vi "LuaVIEW Register Private Function.vi"(5 "LuaVIEW reference in":T1, 7 "function VI path":path, 11 "error in (no error)":errorcluster) -> (6 "LuaVIEW reference out":T1, 15 "error out":errorcluster)   [LabVIEW 2012]
doc: "Open a reference to a LuaVIEW function VI and add it to the LuaVIEW state's private registry so that any script running under that state can call the function."
uses:
  typedefs/t_LuaVIEW Reference.ctl
  typedefs/et_LuaVIEW CIN Actions.ctl
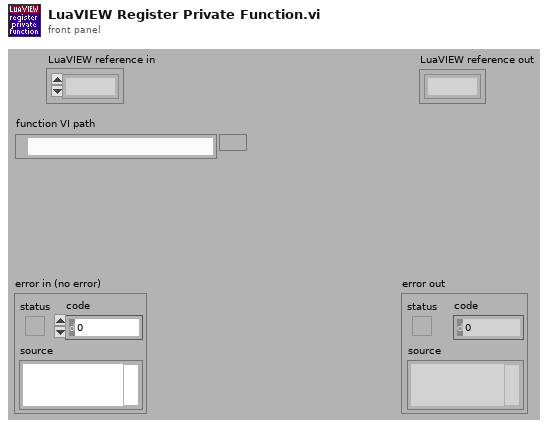
[diagram p1: front panel]
types:
  T1 = typedef "t_LuaVIEW Reference.ctl" = refnum<k1>
  T2 = typedef "et_LuaVIEW CIN Actions.ctl" = enum16{"checksynopsis", "_open", "_registerpublic", "_registerexport", "__never_an_error_result_ns", "luaversion", "cinversion", "_totals", "_taskcount", "pathological", "_unregnextpublic", "registryusecount", "__per_state_actions", "regsetprivate", "regsetindex", "regsetmodule", "_revokeexports", "_usepublic", "prepare", "compile", "execute", "call", "unregstaterefs", "_close", "pullboolean", "pullnumber", "pullI8", "pullU8", "pullI16", "pullU16", "pullI32", "pullU32", "pullobject", "pullrefnum", "pullstring", "pullflat", "pushflat", "pushobject", "getattribute", "setattribute", "stacktostring", "_startyieldtest", "_endyieldtest", "_pollprintbuffer", "__never_an_error_result_ps", "_pollexport", "setclone", "forcecleanup", "gettop", "clearstack", "insert", "pushboolean", "pushnumber", "pushrefnum", "pushstring", "pushnil", "pushvalue", "gettaskref", "settaskref"}
  T3 = typedef "et_LuaVIEW CIN Results.ctl" = enum16{"OK", "error", "main", "call", "clonecall", "modulecall", "exportcall", "index", "yield"}
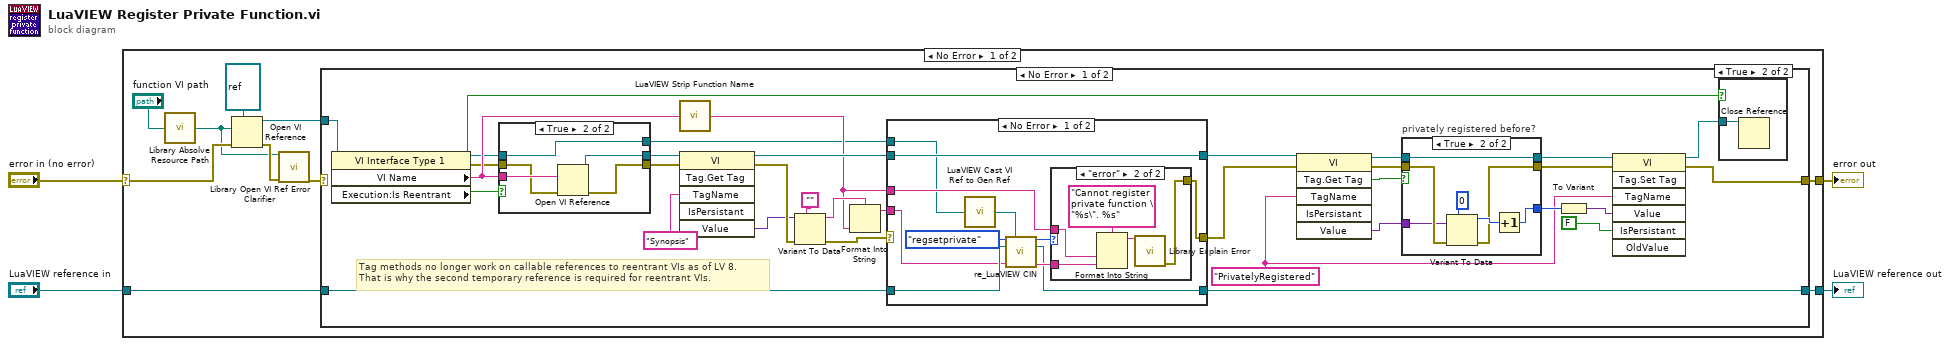
[diagram p0: block diagram]
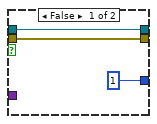
[diagram p4: hidden frame]
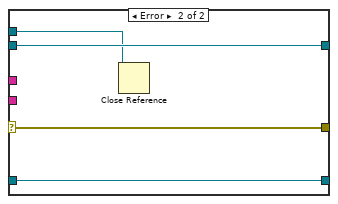
[diagram p6: hidden frame]
diagram:
  n1 = case shown="No Error" "error in (no error)" {
    selector: "error in (no error)" -> [w12 w89]
    tunnel: [w11 w89] -> w4
    tunnel: "LuaVIEW reference in" -> [w10 w88]
    tunnel: [w9 w88] -> w1
    frame No Error {
      n2 = call "Library Absolve Resource Path.vi"("path in"="function VI path") -> ("absolved path"=w7:path)  [unwired: 14 in]
      n3 = Open VI Reference(type specifier VI Refnum (for type only)=refnum<vi> refnum ("function pane"), vi path=w7, error in (no error)=w12) -> (vi reference=w6:refnum<vi>, error out=w8:errorcluster)  [unwired: 3 in]
      n4 = call "Library Open VI Ref Error Clarifier.vi"("VI path"=w7, "called VI error (no error)"=w8) -> ("error out"=w5:errorcluster)  [unwired: 13 in]
      n5 = case shown="No Error" w5 {
        selector: w5 -> [_ w87]
        tunnel: w6 -> [w23 _]
        tunnel: [w16 w87] -> w11
        tunnel: w10 -> [w45 w86]
        tunnel: [w44 w86] -> w9
        frame No Error {
          w35 = "PrivatelyRegistered"
          # "Tag methods no longer work on callable references to reentrant VIs as of LV 8.\nThat is why the second temporary reference is required for reentrant VIs."
          n6 = property class="VI Interface Type 1"(reference=w23) -> (reference out=w18:refnum<vi>, error out=w20:errorcluster, "VI Name"=w22:string, "Execution:Is Reentrant"=w15:bool)  [unwired: 1 in]
          n7 = case shown="True" w15 {
            tunnel: w22 -> [_ w54]
            tunnel: [w48 w53] -> w21
            tunnel: [w49 w51] -> w19
            tunnel: w20 -> [w49 w52]
            tunnel: w18 -> [w48 w50]
            tunnel: [w48 w50] -> w17
            frame False {
            }
            frame True {
              n8 = Open VI Reference(vi path=w54, error in (no error)=w52) -> (vi reference=w53:refnum<vi>, error out=w51:errorcluster)  [unwired: 4 in]
            }
          }
          n9 = call "LuaVIEW Strip Function Name.vi"("function VI name"=w22) -> ("Lua function name"=w24:string)  [unwired: 14 in]
          n10 = invoke class="VI" method="Tag.Get Tag"(reference=w21, error in=w19, "TagName"="Synopsis") -> (reference out=w27:refnum<vi>, error out=w32:errorcluster, "Value"=w28:variant)  [unwired: 3 in, 3 out]
          n11 = Variant To Data(error in=w32, type="", Variant=w28) -> (data=w29:string, error out=w25:errorcluster)
          n12 = Format Into String(format string=w29, w24) -> (resulting string=w26:string)  [unwired: 2 in, 1 out]
          n13 = case shown="No Error" w25 {
            selector: w25 -> [_ w84]
            tunnel: w45 -> [w74 w85]
            tunnel: [w71 w85] -> w44
            tunnel: w27 -> [w67 w83]
            tunnel: w26 -> [w70 _]
            tunnel: w24 -> [w69 _]
            tunnel: [w68 w84] -> w34
            tunnel: [w67 w83] -> w39
            tunnel: w17 -> [w66 w82]
            frame No Error {
              n14 = call "LuaVIEW Cast VI Ref to Gen Ref.vi"("refnum in"=w66) -> ("refnum out"=w75:refnum<vi>)  [unwired: 14 in]
              n15 = call "re_LuaVIEW CIN.vi"("action"=et_LuaVIEW_CIN_Actions."regsetprivate", "refnum in"=w75, "LuaVIEW reference in"=w74, "string in"=w70) -> ("result"=w73:T3, "LuaVIEW reference out"=w71:T1, "string out"=w72:string)  [unwired: 5 in, 4 out]
              n16 = case shown="\"error\"" w73 {
                tunnel: w72 -> [_ w79]
                tunnel: w69 -> [_ w78]
                tunnel: [_ w77] -> w68
                frame Default {
                }
                frame "error" {
                  n17 = Format Into String(format string="Cannot register private function \"%s\". %s", w78, w79) -> (resulting string=w81:string)  [unwired: 2 in, 1 out]
                  n18 = call "Library Explain Error.vi"("explanation prefix (none)"=w81) -> ("explained error"=w77:errorcluster)  [unwired: 14 in]
                }
              }
            }
            frame Error {
              n19 = Close Reference(reference=w82) -> ()  [unwired: 1 in, 1 out]
            }
          }
          n20 = invoke class="VI" method="Tag.Get Tag"(reference=w39, error in=w34, "TagName"=w35) -> (reference out=w40:refnum<vi>, error out=w41:errorcluster, "GetTag"=w43:bool, "Value"=w42:variant)  [unwired: 3 in, 2 out]
          n21 = case "privately registered before?" shown="True" w43 {
            tunnel: w42 -> [_ w63]
            tunnel: w41 -> [w57 w64]
            tunnel: [1 w61] -> w38
            tunnel: [w57 w60] -> w36
            tunnel: w40 -> [w56 w59]
            tunnel: [w56 w59] -> w37
            frame False {
            }
            frame True {
              n22 = Variant To Data(error in=w64, type=0, Variant=w63) -> (data=w62:i32, error out=w60:errorcluster)
              n23 = Increment(x=w62) -> (x+1=w61:i32)
            }
          }
          n24 = To Variant(anything=w38) -> (Variant=w47:variant)
          n25 = invoke class="VI" method="Tag.Set Tag"(reference=w37, error in=w36, "TagName"=w35, "Value"=w47, "IsPersistant"=FALSE) -> (reference out=w33:refnum<vi>, error out=w16:errorcluster)  [unwired: 2 in, 5 out]
          n26 = case shown="True" w15 {
            tunnel: w33 -> [_ w55]
            frame False {
            }
            frame True {
              n27 = Close Reference(reference=w55) -> ()  [unwired: 1 in, 1 out]
            }
          }
        }
        frame Error {
        }
      }
    }
    frame Error {
    }
  }
  "error out" <- w4
  "LuaVIEW reference out" <- w1
